vi "test_read_variable.vi"() -> ()   [LabVIEW 2017]
uses:
  <vilib>/lvdsc/NI_DSC.lvlib
panel:
  out "Array of Double":dbl[][](array[numeric])
  out "Valid?":bool
  out "data":dbl[](array[numeric])
  in  "stop":bool
  out "Numeric":i32
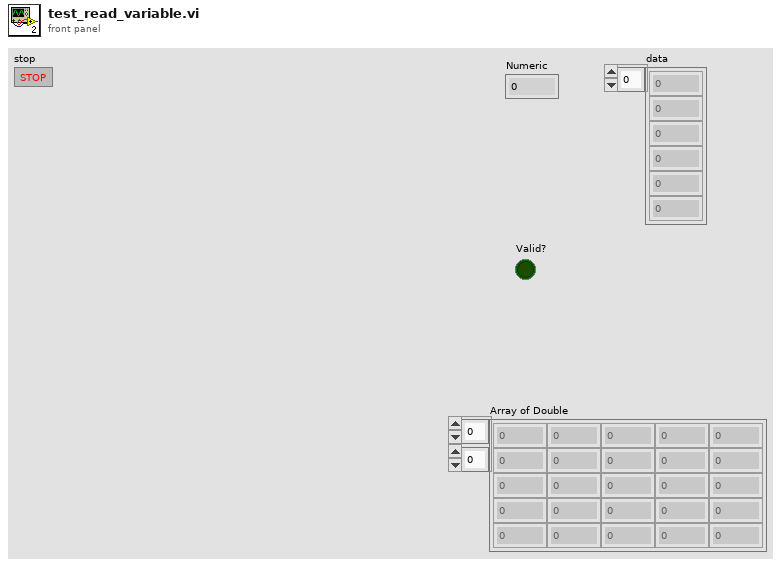
[diagram p1: front panel]
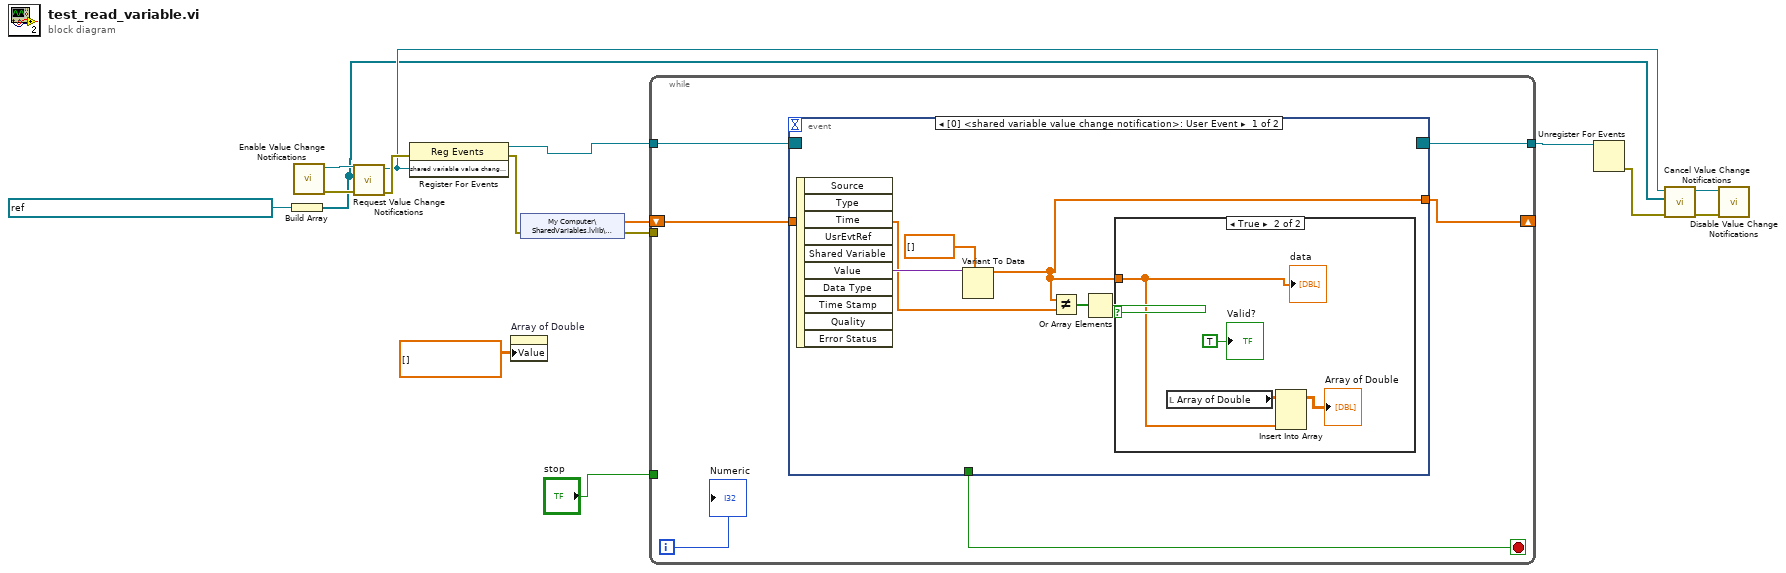
[diagram p0: block diagram]
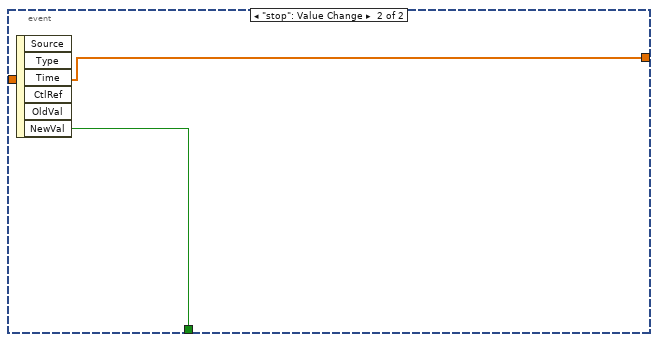
[diagram p3: hidden frame]
diagram:
  n1 = Build Array(refnum<k21> "\\\\My Computer\\SharedVariables\\ImageClick" ("Project Variable Control")) -> (w4:refnum<k21>[])
  n2 = call <vilib>:"Enable Value Change Notifications.vi"() -> ("error out"=w14:errorcluster, "shared variable value change notification"=w15:refnum<user-event>)  [unwired: 10 in]
  n3 = call <vilib>:"Request Value Change Notifications.vi"("error in (no error)"=w14, "shared variables"=w4, "notification refnum"=w15) -> ("error out"=w11:errorcluster, "shared variable value change notification"=w5:refnum<user-event>)  [unwired: 6 in, 1 out]
  n4 = register-events(error in=w11, w5) -> (reference out=w10:refnum<event-registration>, error out=w3:errorcluster)  [unwired: 1 in]
  n5 = property on="Array of Double" class="Arr (strict)"("Value"=dbl[][] [] ("Array of Double")) -> ()  [unwired: 2 in, 2 out]
  n6 = shared-variable "My Computer\\SharedVariables.lvlib\\ImageClick"(error in=w3) -> (w12:dbl[], error out=w2:errorcluster)
  n7 = while {
    tunnel: "stop" -> [_]
    tunnel: w10 -> [w20]
    shift-right: [w18] -> _
    shift-left: w12 -> [w19]
    tunnel: [w17] -> w9
    tunnel: w2 -> [_]
    i -> [w22]
    stop <- w21 stop-if-true
    n8 = event shown="[0] <shared variable value change notification>: User Event" {
      selector: w20 -> [_ _]
      dyn-events: [_ _] -> w17
      timeout: _ -> [_ _]
      tunnel: [_ w34] -> w21
      tunnel: w19 -> [w24 w33]
      tunnel: [w23 w33] -> w18
      event User Event {
        n9 = event-data() -> ("Value"=w28:variant)  [unwired: 1 in, 9 out]
        n10 = Variant To Data(type=dbl[] [], Variant=w28) -> (data=w23:dbl[])  [unwired: 1 in, 1 out]
        n11 = Not Equal?(x=w23, y=w24) -> (x != y?=w26:bool[])
        n12 = Or Array Elements(Boolean array=w26) -> (logical OR=w25:bool)
        n13 = case shown="True" w25 {
          tunnel: w23 -> [_ w29]
          frame False {
          }
          frame True {
            n14 = local read "Array of Double"() -> (w31:dbl[][])
            n15 = Insert Into Array(array=w31, new element=w29) -> (→"Array of Double":dbl[][])  [unwired: 2 in]
            "data" <- w29
            "Valid?" <- TRUE ("Valid?")
          }
        }
      }
      event "stop": Value Change {
        n16 = event-data() -> ("NewVal"=w34:bool)  [unwired: 1 in, 5 out]
      }
    }
    "Numeric" <- w22
  }
  n17 = Unregister For Events(event registration refnum=w9) -> (error out=w6:errorcluster)  [unwired: 1 in]
  n18 = call <vilib>:"Cancel Value Change Notifications.vi"("error in (no error)"=w6, "shared variables"=w4, "notification refnum"=w5) -> ("error out"=w8:errorcluster, "shared variable value change notification"=w7:refnum<user-event>)  [unwired: 6 in, 1 out]
  n19 = call <vilib>:"Disable Value Change Notifications.vi"("error in (no error)"=w8, "notification refnum"=w7) -> ()  [unwired: 9 in, 1 out]
